vi "FPGA Configure Data Buffers.vi"(8 "error in (no error)":errorcluster) -> (0 "error out":errorcluster)   [LabVIEW 2016]
doc: "This vi configures the FPGA FIFO buffers used to transfer raw data to the FPGA and retrieve FFT data from the FPGA."
uses:
  FPGA Global Variables.vi
  <vilib>/rvi/interface/common/niFpgaWaitOnOcc.vi
  <vilib>/Utility/error.llb/Error Cluster From Error Code.vi
  <vilib>/rvi/interface/nirviMethod/nirviMethod.xnode
  <vilib>/FPGAPlugInAG/Dynamic/niLvFpga_ConfigureFifo_Dynamic.vi
  <vilib>/rvi/errors/niLvFpgaMergeErrorWithErrorCode.vi
  <vilib>/FPGAPlugInAG/Dynamic/niLvFpga_StartFifo_Dynamic.vi
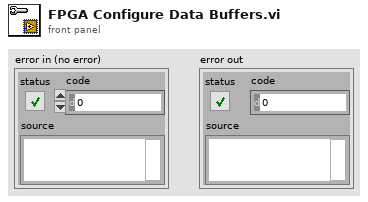
[diagram p1: front panel]
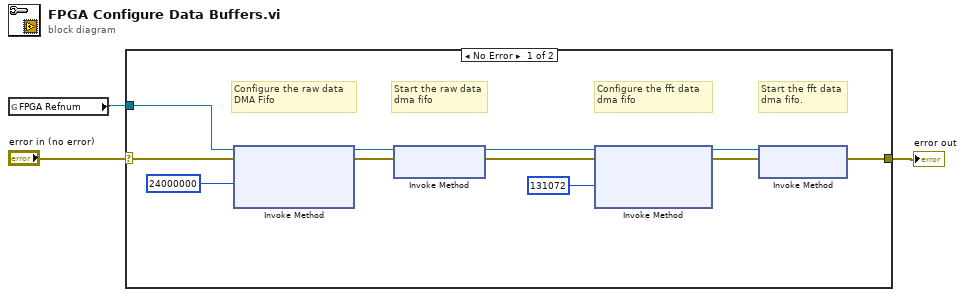
[diagram p0: block diagram]
diagram:
  n1 = global read "FPGA Global Variables.vi" "FPGA Refnum"() -> (w1:refnum<k20>)
  n2 = case shown="No Error" "error in (no error)" {
    selector: "error in (no error)" -> [w6 w15]
    tunnel: w1 -> [w14 _]
    tunnel: [w4 w15] -> w2
    frame No Error {
      # "Start the fft data\ndma fifo."
      # "Configure the fft data\ndma fifo"
      # "Start the raw data\ndma fifo"
      # "Configure the raw data\nDMA Fifo"
      n3 = xnode "Invoke Method"("FPGA VI Reference In"=w14, "error in"=w6, "Requested Depth"=u32 24000000) -> ("FPGA VI Reference Out"=w13:refnum<k20>, "error out"=w12:errorcluster)  [unwired: 1 out]
      n4 = xnode "Invoke Method"("FPGA VI Reference In"=w13, "error in"=w12) -> ("FPGA VI Reference Out"=w11:refnum<k20>, "error out"=w10:errorcluster)
      n5 = xnode "Invoke Method"("FPGA VI Reference In"=w11, "error in"=w10, "Requested Depth"=u32 131072) -> ("FPGA VI Reference Out"=w9:refnum<k20>, "error out"=w8:errorcluster)  [unwired: 1 out]
      n6 = xnode "Invoke Method"("FPGA VI Reference In"=w9, "error in"=w8) -> ("error out"=w4:errorcluster)  [unwired: 1 out]
    }
    frame Error {
    }
  }
  "error out" <- w2
